vi "Temperature Min Read Single.vi"(8 "error in":errorcluster, 9 "Channel Index":i32=1, 11 "Climate Chamber in":refnum<class "Climate Chamber.lvclass">) -> (0 "error out":errorcluster, 1 "Changed or First Call?":bool, 2 "Temperature Min SP":dbl, 3 "Climate Chamber out":refnum<class "Climate Chamber.lvclass">)   [LabVIEW 2023, in "Climate Chamber.lvclass"]
uses:
  Climate Chamber.lvclass
  Low Level Capabilities/Temperature/Temperature Limit/Temperature Limit.lvclass
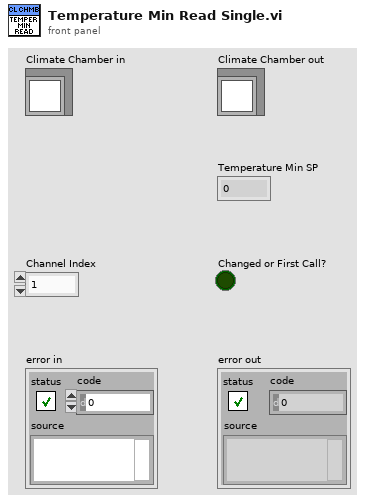
[diagram p1: front panel]
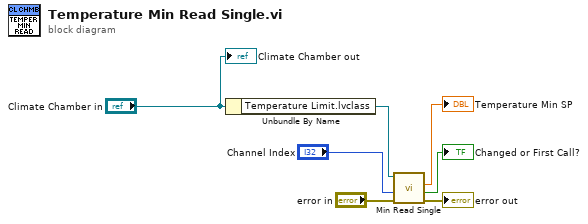
[diagram p0: block diagram]
diagram:
  n1 = Unbundle By Name("Climate Chamber in") -> ("Temperature Limit.lvclass"=w6:refnum<class "Temperature Limit.lvclass">)
  n2 = call-dynamic "Min Read Single.vi"("error in"="error in", "Channel Index"="Channel Index", "Min Temperature Limit in"=w6) -> ("error out"=→"error out":errorcluster, "Changed or First Call?"=→"Changed or First Call?":bool, "Temperature Min SP"=→"Temperature Min SP":dbl)  [unwired: 5 in, 1 out]
  "Climate Chamber out" <- "Climate Chamber in"
